vi "Init.vi"(4 "Y":i32, 6 "X":i32, 11 "Uno in":refnum<class "Uno.lvclass">) -> (3 "Uno out":refnum<class "Uno.lvclass">)   [LabVIEW 2017, in "Uno.lvclass"]
uses:
  Uno.lvclass
  Group Data.ctl
  Uno.lvclass/Uno.ctl
  SubVIs/Read-Only Globals.vi
  SubVIs/Globals (private).vi
  Square/Square.lvclass
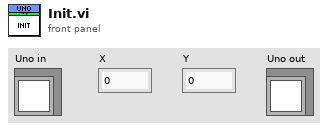
[diagram p1: front panel]
types:
  T1 = typedef "Uno.lvclass/Group Data.ctl" = cluster{"our positions":u8[][]}
  T2 = typedef "Semaphore RefNum" = refnum<k1>
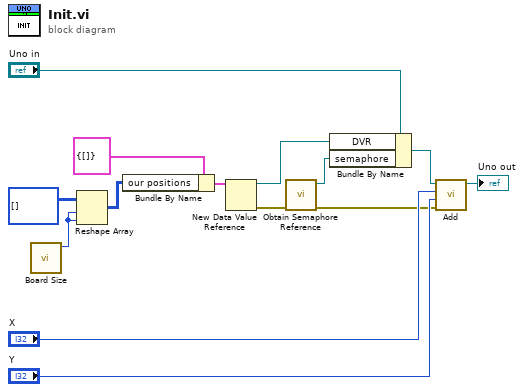
[diagram p0: block diagram]
diagram:
  n1 = call "Board Size.vi"() -> ("Board Size"=w7:i32)  [unwired: 11 in]
  n2 = Reshape Array(u8[][] [] ("our positions"), w7, w7) -> (w8:u8[][])
  n3 = Bundle By Name(cluster=T1 {"our positions"=[]} ("group data"), "our positions"=w8) -> (w11:T1)
  n4 = New Data Value Reference(data value=w11) -> (data value reference=w9:refnum<data-value>, error out=w2:errorcluster)  [unwired: 1 in]
  n5 = call <vilib>:"Obtain Semaphore Reference.vi"("error in (no error)"=w2) -> ("error out"=w1:errorcluster, "semaphore"=w3:T2)  [unwired: 4 in, 1 out]
  n6 = Bundle By Name(cluster="Uno in", "DVR"=w9, "semaphore"=w3) -> (w6:refnum<class "Uno.lvclass">)
  n7 = call "Add.vi"("error in"=w1, "Y"="Y", "X"="X", "Uno in"=w6) -> ("Uno out"=→"Uno out":refnum<class "Uno.lvclass">)  [unwired: 6 in, 1 out]
